vi "New Subset Pointer.vi"(7 "length (-1: rest)":i64=-1 format="%d bytes", 8 "error in (no error)":errorcluster, 9 "offset (0)":u64 format="%d bytes", 10 "subset Pointer type":refnum<class "Pointer.lvclass">, 11 "base Pointer in":refnum<class "Pointer.lvclass">) -> (0 "error out":errorcluster, 1 "offset out":u64 format="%d bytes", 2 "subset Pointer":refnum<class "Pointer.lvclass">, 3 "base Pointer out":refnum<class "Pointer.lvclass">)   [LabVIEW 2017, in "Memory Manager.lvlib" / "Pointer.lvclass"]
uses:
  Pointer.lvclass
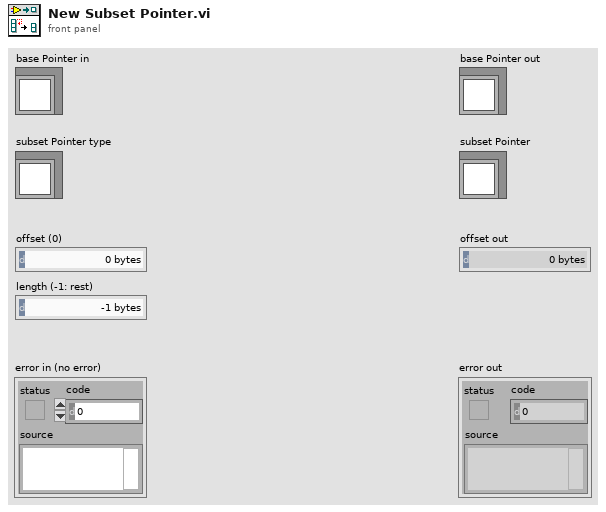
[diagram p1: front panel]
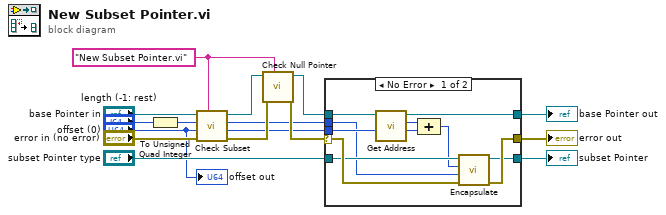
[diagram p0: block diagram]
diagram:
  w3 = "New Subset Pointer.vi" ("source vi name")
  n1 = To Unsigned Quad Integer(1:"length (-1: rest)") -> (0:w12:u64)
  n2 = call "Check Subset.vi"("source vi name"=w3, "error in (no error)"="error in (no error)", "offset (0)"="offset (0)", "length"=w12, "Pointer in"="base Pointer in") -> ("error out"=w16:errorcluster, "offset out"=w6:u64, "length"=w7:u64, "Pointer out"=w5:refnum<class "Pointer.lvclass">)  [unwired: 3 in]
  n3 = call "Check Null Pointer.vi"("source vi name"=w3, "error in (no error)"=w16, "Pointer in"=w5) -> ("error out"=w15:errorcluster, "Pointer out"=w4:refnum<class "Pointer.lvclass">)  [unwired: 7 in]
  n4 = case shown="No Error" w15 {
    selector: w15 -> [w26 w27]
    tunnel: "subset Pointer type" -> [w25 w28]
    tunnel: [w23 w28] -> w9
    tunnel: w4 -> [w22 w29]
    tunnel: [w21 w29] -> w8
    tunnel: w7 -> [w17 _]
    tunnel: w6 -> [w20 _]
    tunnel: [w24 w27] -> w2
    frame No Error {
      n5 = call "Get Address.vi"("Pointer in"=w22) -> ("address"=w19:u64, "Pointer out"=w21:refnum<class "Pointer.lvclass">)  [unwired: 9 in]
      n6 = Compound Arithmetic op=ADD(w19, w20) -> (w18:u64)
      n7 = call "Encapsulate.vi"("error in (no error)"=w26, "size"=w17, "address"=w18, "Pointer type"=w25) -> ("error out"=w24:errorcluster, "Pointer out"=w23:refnum<class "Pointer.lvclass">)  [unwired: 6 in]
    }
    frame Error {
    }
  }
  "error out" <- w2
  "subset Pointer" <- w9
  "base Pointer out" <- w8
  "offset out" <- "offset (0)"
